vi "DetecElec外观.vi"(0 "Data In":T3 caption="数据输入", 2 "Display State In":T2 caption="显示状态输入", 3 "Container State":T4 caption="容器状态") -> (6 "Data Out":T3 caption="数据输出", 7 "Display State Out":T2 caption="显示状态输出", 8 "Action":T1 caption="动作")   [LabVIEW 2014, in "DetecElecXControl.xctl"]
uses:
  DetecElecXControl.xctl
  <vilib>/_xctls/Container State.ctl
  <vilib>/_xctls/Action.ctl
  <vilib>/_xctls/XControlSupport.lvlib
panel:
  out "VV":string
  out "MapY":string
  out "MapX":string
  out "elename":string
  out "ele":bool
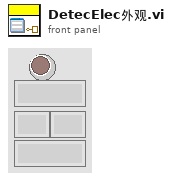
[diagram p1: front panel]
types:
  T1 = typedef "XControlSupport.lvlib/Action.ctl" = cluster{"Data Changed?":bool, "State Changed?":bool, "Action Name":string}
  T2 = typedef "DetecElecXControl.xctl/DetecElec状态.ctl" = cluster{"是否显示":bool, "Ele":T3}
  T3 = typedef "DetecElecXControl.xctl/DetecElec数据.ctl" = cluster{"Data":bool, "ElecName":string, "mapX":string, "mapY":string, "VV":string}
  T4 = typedef "XControlSupport.lvlib/Container State.ctl" = cluster{"Indicator?":bool, "Run Mode?":bool, " Refnum":refnum<vi>}
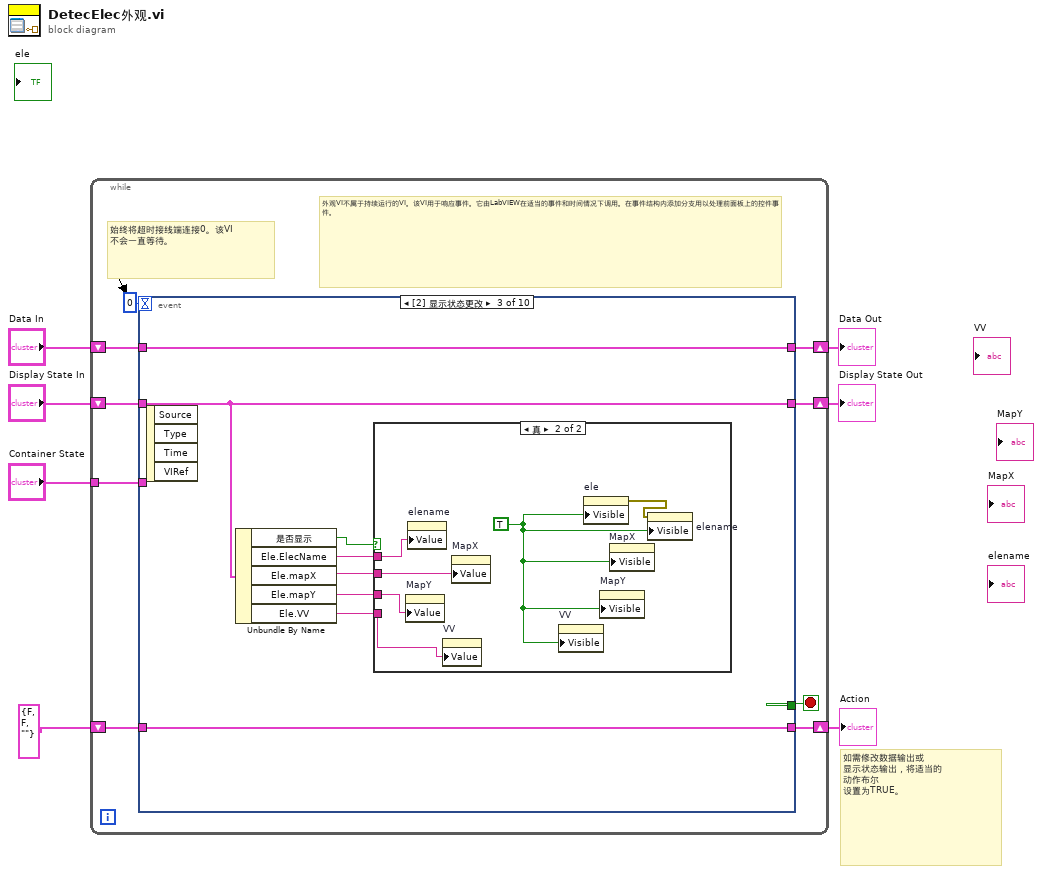
[diagram p0: block diagram]
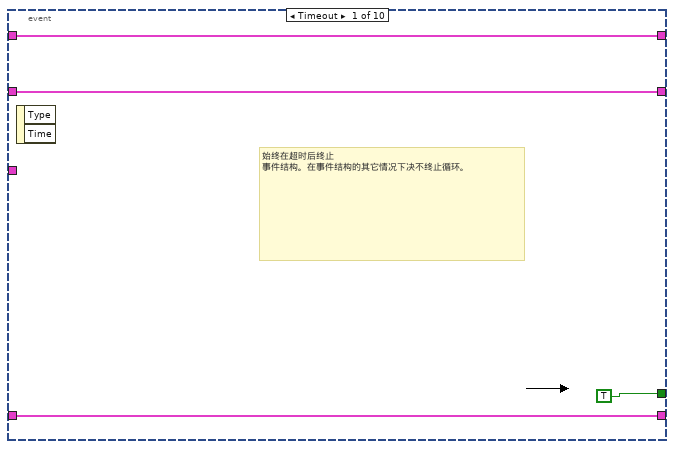
[diagram p2: hidden frame]
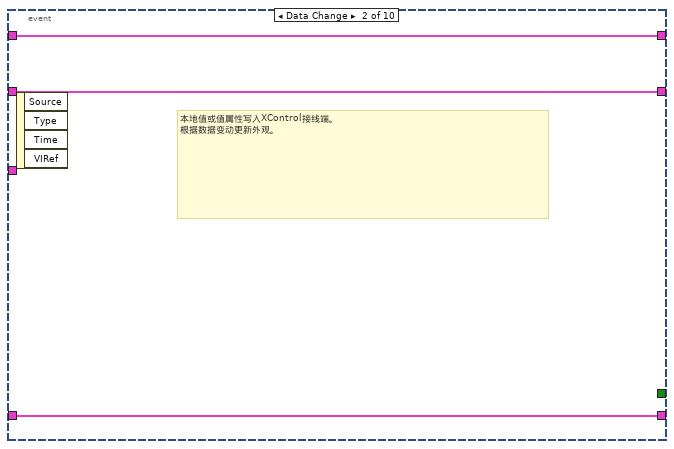
[diagram p3: hidden frame]
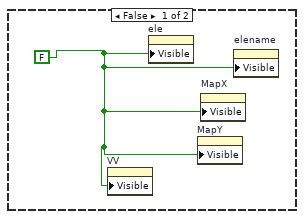
[diagram p4: hidden frame]
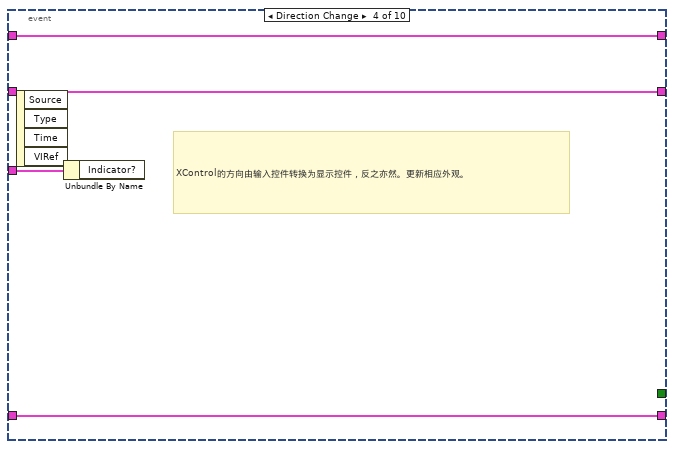
[diagram p5: hidden frame]
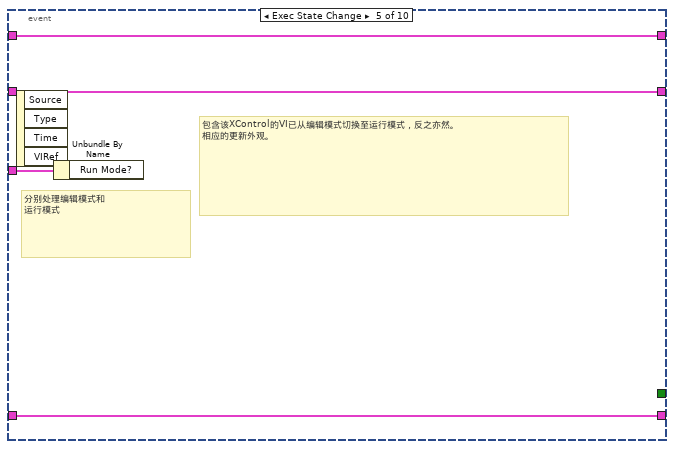
[diagram p6: hidden frame]
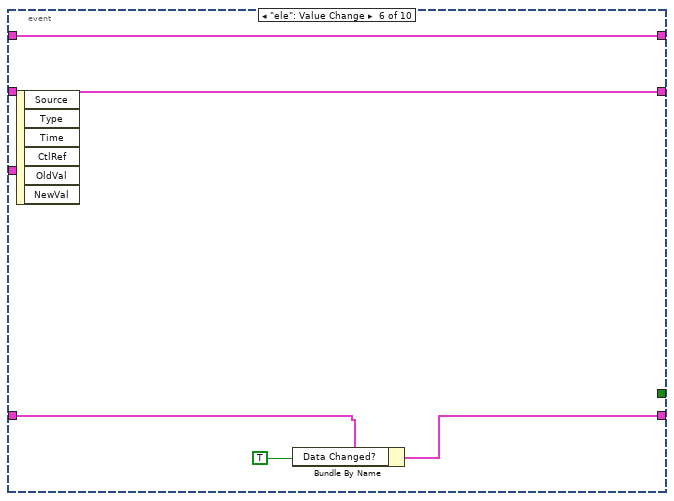
[diagram p7: hidden frame]
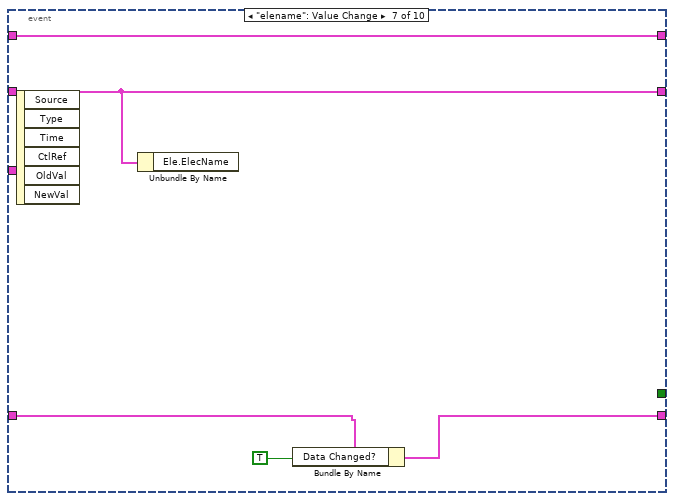
[diagram p8: hidden frame]
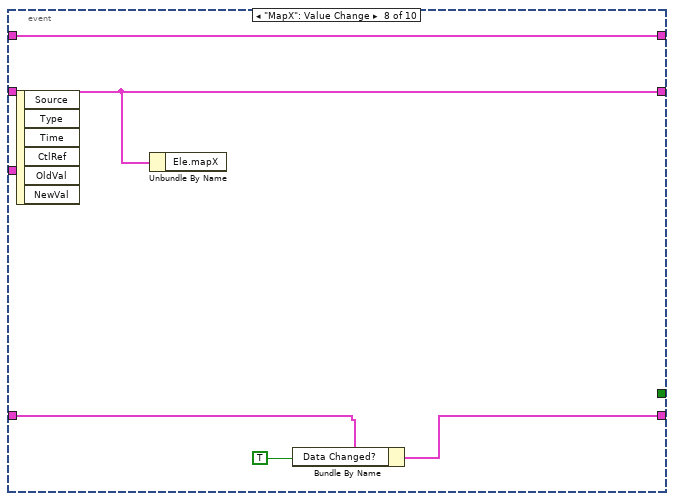
[diagram p9: hidden frame]
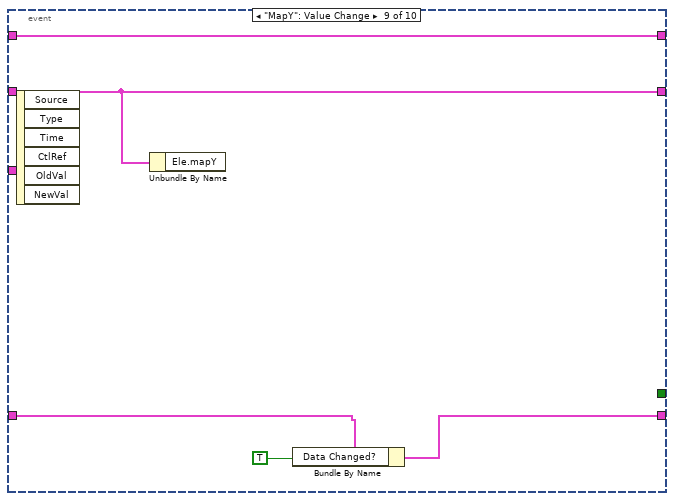
[diagram p10: hidden frame]
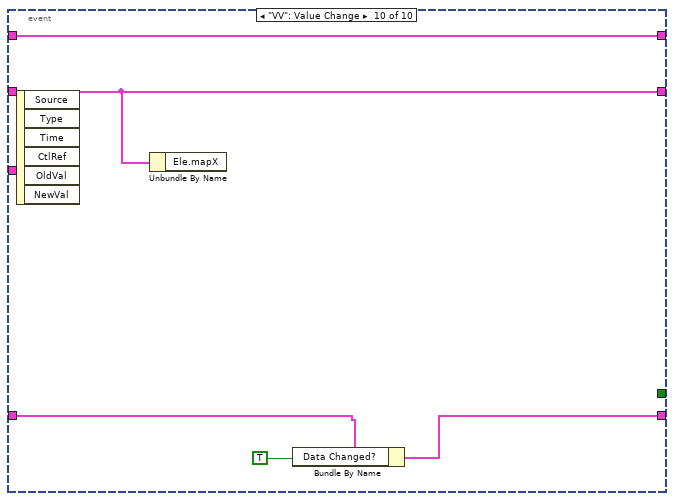
[diagram p11: hidden frame]
diagram:
  # "如需修改数据输出或\n显示状态输出，将适当的\n动作布尔\n设置为TRUE。"
  n1 = while {
    shift-right: [w15] -> w4
    shift-left: "Display State In" -> [w16]
    tunnel: "Container State" -> [w12]
    shift-right: [w10] -> w7
    shift-left: "Data In" -> [w11]
    shift-right: [w8] -> w2
    shift-left: T1 {"Data Changed?"=FALSE, "State Changed?"=FALSE, "Action Name"=""} ("Action") -> [w9]
    stop <- w14 stop-if-true
    # "外观VI不属于持续运行的VI。该VI用于响应事件。它由LabVIEW在适当的事件和时间情况下调用。在事件结构内添加分支用以处理前面板上的控件事件。"
    # "始终将超时接线端连接0。该VI\n不会一直等待。"
    n2 = event shown="[2] 显示状态更改" {
      selector: _ -> [_ _ _ _ _ _ _ _ _ _]
      dyn-events: _ -> [_ _ _ _ _ _ _ _ _ _]
      timeout: 0 -> [_ _ _ _ _ _ _ _ _ _]
      tunnel: w16 -> [w18 w22 w29 w41 w45 w51 w52 w57 w62 w67]
      tunnel: [w18 w22 w29 w41 w45 w51 w52 w57 w62 w67] -> w15
      tunnel: [TRUE _ _ _ _ _ _ _ _ _] -> w14
      tunnel: w12 -> [_ _ _ w42 w46 _ _ _ _ _]
      tunnel: w11 -> [w17 w23 w31 w40 w44 w50 w56 w61 w66 w71]
      tunnel: [w17 w23 w31 w40 w44 w50 w56 w61 w66 w71] -> w10
      tunnel: [w19 w21 w30 w39 w43 w47 w53 w58 w63 w68] -> w8
      tunnel: w9 -> [w19 w21 w30 w39 w43 w48 w54 w59 w64 w69]
      event Timeout {
        # "始终在超时后终止\n事件结构。在事件结构的其它情况下决不终止循环。"
        n3 = event-data() -> ()  [unwired: 1 in, 2 out]
      }
      event Data Change {
        # "本地值或值属性写入XControl接线端。\n根据数据变动更新外观。"
        n4 = event-data() -> ()  [unwired: 1 in, 4 out]
      }
      event Display State Change {
        n5 = event-data() -> ()  [unwired: 1 in, 4 out]
        n6 = Unbundle By Name(w29) -> ("是否显示"=w28:bool, "Ele.ElecName"=w26:string, "Ele.mapX"=w25:string, "Ele.mapY"=w24:string, "Ele.VV"=w27:string)
        n7 = case shown="真" w28 {
          tunnel: w27 -> [_ w36]
          tunnel: w26 -> [_ w35]
          tunnel: w25 -> [_ w34]
          tunnel: w24 -> [_ w33]
          frame False {
            w32 = FALSE
            n8 = property on="VV" class="Str"("Visible"=w32) -> ()  [unwired: 2 in, 2 out]
            n9 = property on="ele" class="Bool (严格)"("Visible"=w32) -> ()  [unwired: 2 in, 2 out]
            n10 = property on="MapY" class="Str"("Visible"=w32) -> ()  [unwired: 2 in, 2 out]
            n11 = property on="MapX" class="Str"("Visible"=w32) -> ()  [unwired: 2 in, 2 out]
            n12 = property on="elename" class="Str"("Visible"=w32) -> ()  [unwired: 2 in, 2 out]
          }
          frame True {
            w37 = TRUE
            n13 = property on="MapY" class="Str"("Value"=w33) -> ()  [unwired: 2 in, 2 out]
            n14 = property on="elename" class="Str"("Value"=w35) -> ()  [unwired: 2 in, 2 out]
            n15 = property on="VV" class="Str"("Value"=w36) -> ()  [unwired: 2 in, 2 out]
            n16 = property on="MapX" class="Str"("Value"=w34) -> ()  [unwired: 2 in, 2 out]
            n17 = property on="VV" class="Str"("Visible"=w37) -> ()  [unwired: 2 in, 2 out]
            n18 = property on="ele" class="Bool (严格)"("Visible"=w37) -> (error out=w38:errorcluster)  [unwired: 2 in, 1 out]
            n19 = property on="MapY" class="Str"("Visible"=w37) -> ()  [unwired: 2 in, 2 out]
            n20 = property on="MapX" class="Str"("Visible"=w37) -> ()  [unwired: 2 in, 2 out]
            n21 = property on="elename" class="Str"(error in=w38, "Visible"=w37) -> ()  [unwired: 1 in, 2 out]
          }
        }
      }
      event Direction Change {
        # "XControl的方向由输入控件转换为显示控件，反之亦然。更新相应外观。"
        n22 = event-data() -> ()  [unwired: 1 in, 4 out]
        n23 = Unbundle By Name(w42) -> ()  [unwired: 1 out]
      }
      event Exec State Change {
        # "包含该XControl的VI已从编辑模式切换至运行模式，反之亦然。\n相应的更新外观。"
        # "分别处理编辑模式和\n运行模式"
        n24 = event-data() -> ()  [unwired: 1 in, 4 out]
        n25 = Unbundle By Name(w46) -> ()  [unwired: 1 out]
      }
      event "ele": Value Change {
        n26 = event-data() -> ()  [unwired: 1 in, 6 out]
        n27 = Bundle By Name(cluster=w48, "Data Changed?"=TRUE) -> (w47:T1)
      }
      event "elename": Value Change {
        n28 = event-data() -> ()  [unwired: 1 in, 6 out]
        n29 = Unbundle By Name(w52) -> ()  [unwired: 1 out]
        n30 = Bundle By Name(cluster=w54, "Data Changed?"=TRUE) -> (w53:T1)
      }
      event "MapX": Value Change {
        n31 = event-data() -> ()  [unwired: 1 in, 6 out]
        n32 = Unbundle By Name(w57) -> ()  [unwired: 1 out]
        n33 = Bundle By Name(cluster=w59, "Data Changed?"=TRUE) -> (w58:T1)
      }
      event "MapY": Value Change {
        n34 = event-data() -> ()  [unwired: 1 in, 6 out]
        n35 = Unbundle By Name(w62) -> ()  [unwired: 1 out]
        n36 = Bundle By Name(cluster=w64, "Data Changed?"=TRUE) -> (w63:T1)
      }
      event "VV": Value Change {
        n37 = event-data() -> ()  [unwired: 1 in, 6 out]
        n38 = Unbundle By Name(w67) -> ()  [unwired: 1 out]
        n39 = Bundle By Name(cluster=w69, "Data Changed?"=TRUE) -> (w68:T1)
      }
    }
  }
  "Display State Out" <- w4
  "Data Out" <- w7
  "Action" <- w2
